vi "EtherSerialComms.vi"(6 "byteCount":i32, 7 "mode":T1(ring)=enum."CRLF", 9 "Timeout/ms":u32, 10 "Write":string, 11 "Port Name":string) -> (0 "error out":errorcluster, 2 "commsTime(s)":dbl, 3 "data out":string)   [LabVIEW 2021]
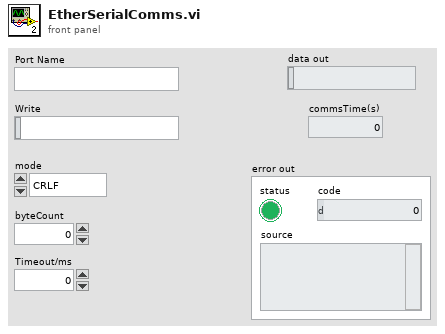
[diagram p1: front panel]
types:
  T1 = enum16{"Standard", "Buffered", "CRLF", "Immediate"}
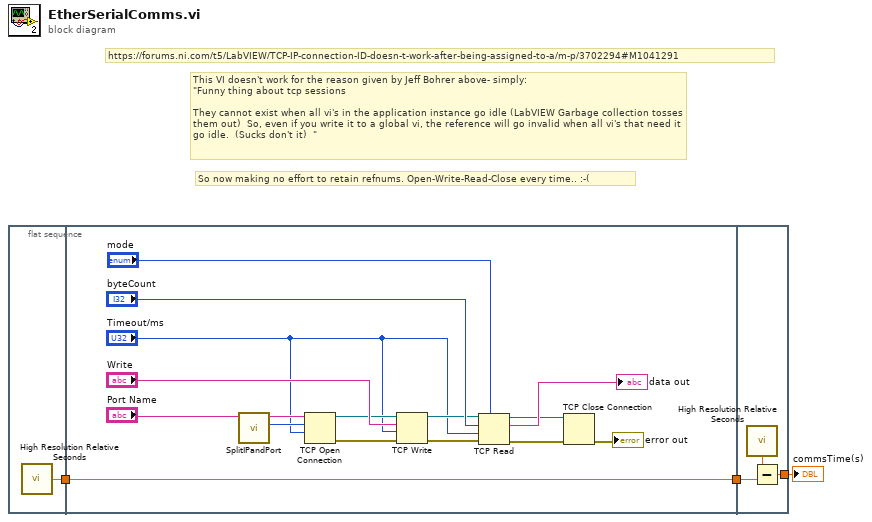
[diagram p0: block diagram]
diagram:
  # "So now making no effort to retain refnums. Open-Write-Read-Close every time.. :-("
  # "This VI doesn't work for the reason given by Jeff Bohrer above- simply:\n\"Funny thing about tcp sessions\n \nThey cannot exist when all vi's in the application instance go idle (LabVIEW Garbage collection tosses them out)  So, even if you write it to a global vi, the reference will go invalid when all vi's that need it go idle.  (Sucks don't it)  \""
  # "https://forums.ni.com/t5/LabVIEW/TCP-IP-connection-ID-doesn-t-work-after-being-assigned-to-a/m-p/3702294#M1041291"
  n1 = flat-sequence {
    tunnel: [w4] -> w3
    tunnel: w3 -> [w5]
    tunnel: [w5] -> w2
    tunnel: w2 -> [w22]
    tunnel: [w21] -> w1
    frame #0 {
      n2 = call <vilib>:"High Resolution Relative Seconds.vi"() -> ("relative seconds"=w4:dbl)
    }
    frame #1 {
      n3 = call "SplitIPandPort.vi"("IP:Port"="Port Name") -> ("Port"=w17:u16, "IP"=w16:string)  [unwired: 9 in]
      n4 = TCP Open Connection(address=w16, remote port or service name=w17, timeout ms (60000)="Timeout/ms") -> (connection ID=w10:refnum<k5>, error out=w11:errorcluster)  [unwired: 2 in]
      n5 = TCP Write(connection ID=w10, data in="Write", error in (no error)=w11, 9:"Timeout/ms") -> (connection ID out=w14:refnum<k5>, error out=w15:errorcluster)  [unwired: 1 out]
      n6 = TCP Read(connection ID=w14, bytes to read="byteCount", error in (no error)=w15, 7:"mode", 9:"Timeout/ms") -> (connection ID out=w9:refnum<k5>, data out=→"data out":string, error out=w8:errorcluster)
      n7 = TCP Close Connection(connection ID=w9, error in (no error)=w8) -> (error out=→"error out":errorcluster)  [unwired: 1 in, 1 out]
    }
    frame #2 {
      n8 = call <vilib>:"High Resolution Relative Seconds.vi"() -> ("relative seconds"=w23:dbl)
      n9 = Subtract(x=w23, y=w22) -> (x-y=w21:dbl)
    }
  }
  "commsTime(s)" <- w1
